vi "Color-Roulette.vi"(11 "Color":string="Other") -> (3 "On It":bool)   [LabVIEW 2019]
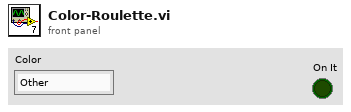
[diagram p1: front panel]
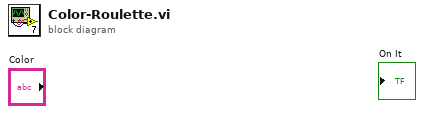
[diagram p0: block diagram]
diagram:
